vi "Predict size from GB DoF.vi"(8 "Integer Tolerance":dbl=0.05, 9 "Lattice Parameter":dbl=6.615785553057252, 10 "Mutual Viewing Angle":dbl[](array[numeric])=[0.0, 1.0, 0.0], 11 "Grain Boundary Definition":T2={"Grain 1 Orientation"=[1.0, 1.0, 1.0], "Grain 2 Orientation"=[1.0, 1.0, 1.0], "Twist Angle (Deg)"=60.0, "Translation Vector"=[0.0, 0.0, 0.0]}) -> (1 "# of Atoms":i32, 2 "Expected Volume (A3)":dbl, 3 "Suggested Dimensions":T1)   [LabVIEW 2010]
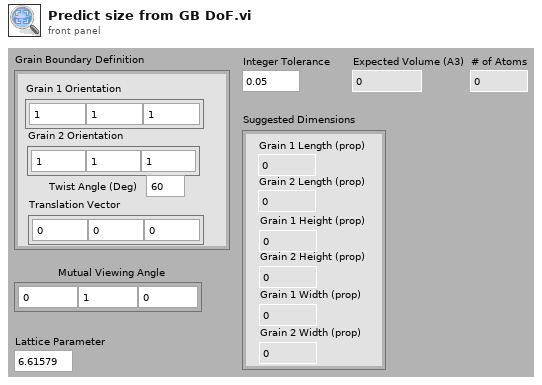
[diagram p1: front panel]
types:
  T1 = cluster{"Grain 1 Length (prop)":dbl, "Grain 2 Length (prop)":dbl, "Grain 1 Height (prop)":dbl, "Grain 2 Height (prop)":dbl, "Grain 1 Width (prop)":dbl, "Grain 2 Width (prop)":dbl}
  T2 = cluster{"Grain 1 Orientation":dbl[], "Grain 2 Orientation":dbl[], "Twist Angle (Deg)":dbl, "Translation Vector":dbl[]}
  T3 = cluster{"Grain 1 Orientation":dbl[], "Grain 2 Orientation":dbl[], "Twist Angle (Deg)":dbl}
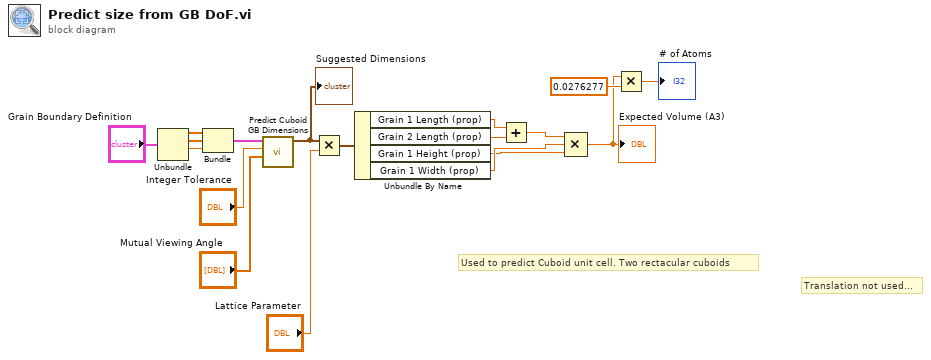
[diagram p0: block diagram]
diagram:
  # "Used to predict Cuboid unit cell. Two rectacular cuboids"
  # "Translation not used..."
  n1 = Unbundle("Grain Boundary Definition") -> ("Grain 1 Orientation"=w7:dbl[], "Grain 2 Orientation"=w6:dbl[], "Twist Angle (Deg)"=w5:dbl)  [unwired: 1 out]
  n2 = Bundle("Grain 1 Orientation"=w7, "Grain 2 Orientation"=w6, "Twist Angle (Deg)"=w5) -> (w4:T3)  [unwired: 1 in]
  n3 = call "Predict Cuboid GB Dimensions.vi"("Mutual Viewing Angle"="Mutual Viewing Angle", "Tolerance"="Integer Tolerance", "Grain Boundary Macro Definition"=w4) -> ("Suggested Cuboid Dimensions (proportional)"=w3:T1)  [unwired: 6 in, 2 out]
  "Suggested Dimensions" <- w3
  n4 = Multiply(x=w3, y="Lattice Parameter") -> (x*y=w1:T1)
  n5 = Unbundle By Name(w1) -> ("Grain 1 Length (prop)"=w13:dbl, "Grain 2 Length (prop)"=w12:dbl, "Grain 1 Height (prop)"=w10:dbl, "Grain 1 Width (prop)"=w11:dbl)
  n6 = Add(x=w13, y=w12) -> (x+y=w17:dbl)
  n7 = Compound Arithmetic op=MULTIPLY(w17, w11, w10) -> (w15:dbl)
  "Expected Volume (A3)" <- w15
  n8 = Multiply(x=w15, y=0.0276277) -> (x*y=→"# of Atoms":dbl)
